vi "TagWrite.vi"(7 "LabVIEW Web Service Request":refnum<class "Web Request.lvclass">, 10 "tagName":string, 11 "type":string) -> ()   [LabVIEW 2013]
doc: "TagWrite assigns the given value to the tag specified. Specifying the type isn't required, but results in slightly faster performance."
uses:
  <vilib>/wsapi/Web Request.lvclass
  <vilib>/NI/Tag Bus/tag/Data Type.ctl
  <vilib>/NI/Tag Bus/table/data polymorphs/write one/write Double.vi
  <vilib>/NI/Tag Bus/table/data polymorphs/write one/write Single.vi
  <vilib>/NI/Tag Bus/table/data polymorphs/write one/write I64.vi
  <vilib>/NI/Tag Bus/table/data polymorphs/write one/write I32.vi
  <vilib>/NI/Tag Bus/table/data polymorphs/write one/write I16.vi
  <vilib>/NI/Tag Bus/table/data polymorphs/write one/write I8.vi
  <vilib>/NI/Tag Bus/table/data polymorphs/write one/write U64.vi
  <vilib>/NI/Tag Bus/table/data polymorphs/write one/write U32.vi
  <vilib>/NI/Tag Bus/table/data polymorphs/write one/write U16.vi
  <vilib>/NI/Tag Bus/table/data polymorphs/write one/write U8.vi
  <vilib>/NI/Tag Bus/table/data polymorphs/write one/write String.vi
  <vilib>/NI/Tag Bus/table/data polymorphs/write one/write Boolean.vi
  <vilib>/NI/TagWebClient/API/tagweb client API.lvlib
  <vilib>/NI/Tag Bus/tag/tag descriptor.lvclass
  <vilib>/NI/Tag Bus/table/data table.lvlib
  <vilib>/NI/Tag Bus/dictionary/data dictionary.lvclass
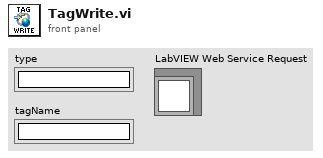
[diagram p1: front panel]
types:
  T1 = typedef "tag bus.lvlib/tag descriptor.lvclass/Data Type.ctl" = enum16{"Double", "Single", "I64", "I32", "I16", "I8", "U64", "U32", "U16", "U8", "Boolean", "String", "Array of Double", "Array of Single", "Array of I64", "Array of I32", "Array of I16", "Array of I8", "Array of U64", "Array of U32", "Array of U16", "Array of U8", "Array of Boolean", "Array of String"}
  T2 = typedef "tag bus.lvlib/data table.lvlib/data table.ctl" = cluster{"Double":dbl[], "Single":sgl[], "I64":i64[], "I32":i32[], "I16":i16[], "I8":i8[], "U64":u64[], "U32":u32[], "U16":u16[], "U8":u8[], "Boolean":bool[], "String":string[], "Array of Double":cluster{"DBL Array":dbl[]}[], "Array of Single":cluster{"SGL Array":sgl[]}[], "Array of I64":cluster{"I64 Array":i64[]}[], "Array of I32":cluster{"I32 Array":i32[]}[], "Array of I16":cluster{"I16 Array":i16[]}[], "Array of I8":cluster{"I8 Array":i8[]}[], "Array of U64":cluster{"U64 Array":u64[]}[], "Array of U32":cluster{"U32 Array":u32[]}[], "Array of U16":cluster{"U16 Array":u16[]}[], "Array of U8":cluster{"U8 Array":u8[]}[], "Array of Boolean":cluster{"Boolean Array":bool[]}[], "Array of String":cluster{"String Array":string[]}[]}
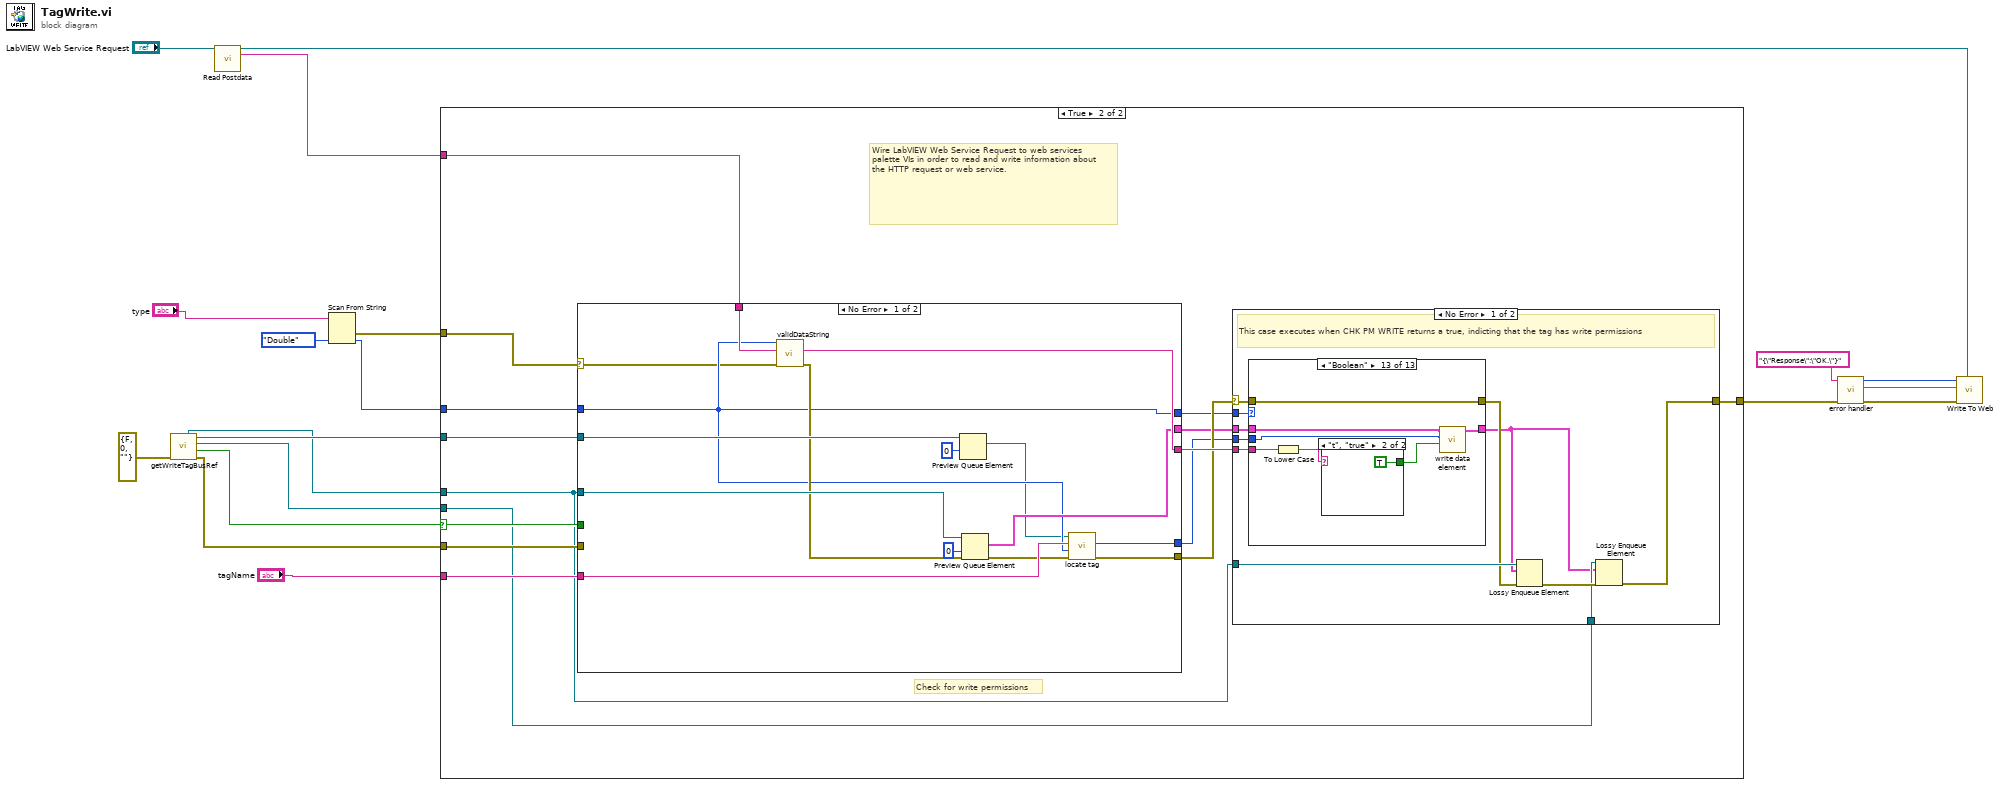
[diagram p0: block diagram]
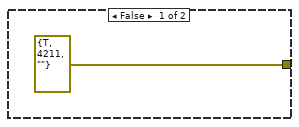
[diagram p2: hidden frame]
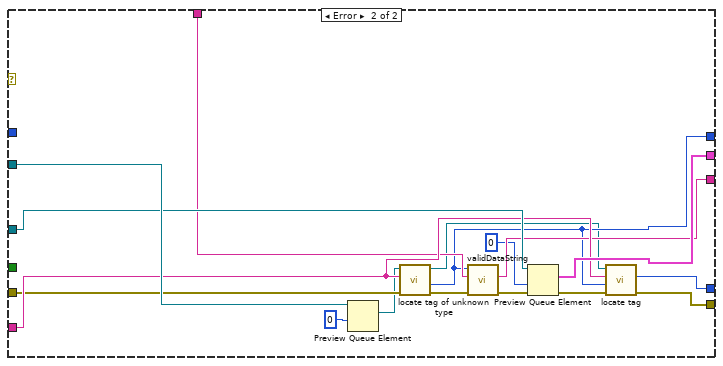
[diagram p3: hidden frame]
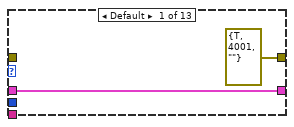
[diagram p4: hidden frame]
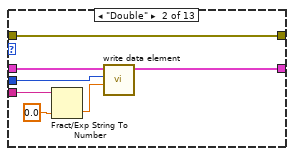
[diagram p5: hidden frame]
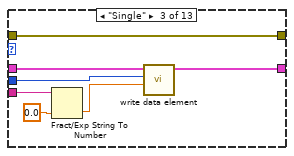
[diagram p6: hidden frame]
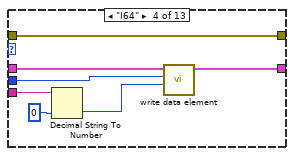
[diagram p7: hidden frame]
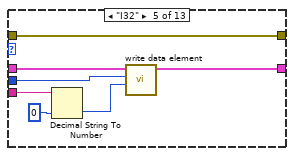
[diagram p8: hidden frame]
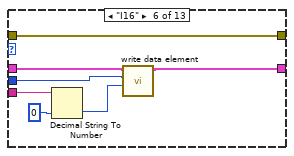
[diagram p9: hidden frame]
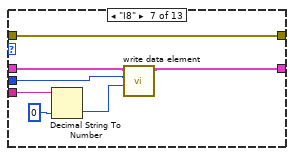
[diagram p10: hidden frame]
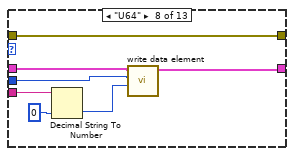
[diagram p11: hidden frame]
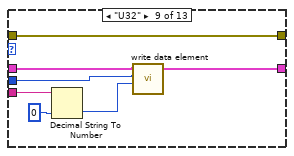
[diagram p12: hidden frame]
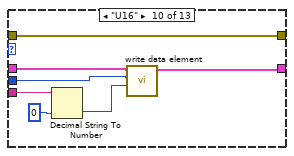
[diagram p13: hidden frame]
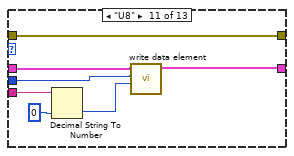
[diagram p14: hidden frame]
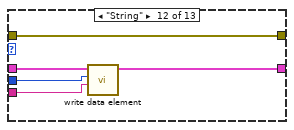
[diagram p15: hidden frame]
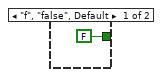
[diagram p16: hidden frame]
diagram:
  n1 = call "getWriteTagBusRef.vi"("error in"=errorcluster {"status"=FALSE, "code"=0, "source"=""} ("error in (no error)")) -> ("error out"=w14:errorcluster, "valid references"=w5:bool, "write tx data table"=w9:refnum<queue>, "write data dictionary"=w15:refnum<queue>, "actual write data table"=w10:refnum<queue>)  [unwired: 6 in]
  n2 = call <vilib>:"Read Postdata.vi"("LabVIEW Web Service Request"="LabVIEW Web Service Request") -> ("LabVIEW Web Service Request out"=w1:refnum<class "Web Request.lvclass">, "postdata"=w4:string)  [unwired: 12 in, 1 out]
  n3 = Scan From String(input string="type", default 1=Data_Type."Double" ("data type")) -> (error out=w12:errorcluster, output 1=w11:T1)  [unwired: 3 in, 2 out]
  n4 = case shown="True" w5 {
    selector: w5 -> [_ w23]
    tunnel: [errorcluster {"status"=TRUE, "code"=4211, "source"=""} ("error IO") w35] -> w18
    tunnel: w15 -> [_ w34]
    tunnel: w14 -> [_ w28]
    tunnel: w4 -> [_ w27]
    tunnel: "tagName" -> [_ w26]
    tunnel: w12 -> [_ w25]
    tunnel: w11 -> [_ w24]
    tunnel: w10 -> [_ w21]
    tunnel: w9 -> [_ w22]
    frame False {
    }
    frame True {
      # "Check for write permissions"
      # "Wire LabVIEW Web Service Request to web services palette VIs in order to read and write information about the HTTP request or web service."
      n5 = case shown="No Error" w25 {
        selector: w25 -> [w36 _]
        tunnel: w27 -> [w50 w61]
        tunnel: w34 -> [w49 w67]
        tunnel: w21 -> [w48 w66]
        tunnel: [w47 w60] -> w33
        tunnel: w23 -> [_ _]
        tunnel: w26 -> [w45 w62]
        tunnel: [w44 w65] -> w32
        tunnel: [w41 w59] -> w31
        tunnel: [w43 w64] -> w30
        tunnel: [w42 w63] -> w29
        tunnel: w28 -> [_ w58]
        tunnel: w24 -> [w41 _]
        frame No Error {
          n6 = call "validDataString.vi"("error in (no error)"=w36, "value in"=w50, "data type"=w41) -> ("error out"=w46:errorcluster, "value out"=w47:string)  [unwired: 6 in, 1 out]
          n7 = Preview Queue Element(queue=w49, timeout in ms (-1)=0) -> (element=w37:refnum<class "data dictionary.lvclass">)  [unwired: 1 in, 3 out]
          n8 = Preview Queue Element(queue=w48, timeout in ms (-1)=0, error in (no error)=w46) -> (element=w42:T2, error out=w39:errorcluster)  [unwired: 2 out]
          n9 = call <vilib>:"locate tag.vi"("error in"=w39, "data type"=w41, "name"=w45, "data dictionary in"=w37) -> ("error out"=w44:errorcluster, "index"=w43:i32)  [unwired: 5 in, 1 out]
        }
        frame Error {
          n10 = Preview Queue Element(queue=w67, timeout in ms (-1)=0) -> (element=w51:refnum<class "data dictionary.lvclass">)  [unwired: 1 in, 3 out]
          n11 = call <vilib>:"locate tag of unknown type.vi"("error in"=w58, "name"=w62, "data dictionary in"=w51) -> ("error out"=w53:errorcluster, "data type"=w59:T1, "data dictionary out"=w52:refnum<class "data dictionary.lvclass">)  [unwired: 5 in, 1 out]
          n12 = call "validDataString.vi"("error in (no error)"=w53, "value in"=w61, "data type"=w59) -> ("error out"=w54:errorcluster, "value out"=w60:string)  [unwired: 6 in, 1 out]
          n13 = Preview Queue Element(queue=w66, timeout in ms (-1)=0, error in (no error)=w54) -> (element=w63:T2, error out=w56:errorcluster)  [unwired: 2 out]
          n14 = call <vilib>:"locate tag.vi"("error in"=w56, "data type"=w59, "name"=w62, "data dictionary in"=w52) -> ("error out"=w65:errorcluster, "index"=w64:i32)  [unwired: 5 in, 1 out]
        }
      }
      n15 = case shown="No Error" w32 {
        selector: w32 -> [w74 w165]
        tunnel: w33 -> [w78 _]
        tunnel: w30 -> [w77 _]
        tunnel: [w70 w165] -> w35
        tunnel: w31 -> [w76 _]
        tunnel: w29 -> [w75 _]
        tunnel: w21 -> [w73 _]
        tunnel: w22 -> [w69 _]
        frame No Error {
          # "This case executes when CHK PM WRITE returns a true, indicting that the tag has write permissions"
          n16 = case shown="\"Boolean\"" w76 {
            tunnel: w77 -> [_ w84 w89 w96 w103 w110 w117 w125 w132 w138 w145 w153 w157]
            tunnel: [errorcluster {"status"=TRUE, "code"=4001, "source"=""} ("error out") w82 w92 w99 w106 w113 w120 w127 w134 w141 w148 w155 w160] -> w72
            tunnel: w78 -> [_ w87 w94 w101 w108 w115 w122 w129 w136 w143 w150 w152 w162]
            tunnel: w75 -> [w79 w85 w91 w98 w104 w111 w118 w126 w133 w140 w146 w154 w159]
            tunnel: w74 -> [_ w82 w92 w99 w106 w113 w120 w127 w134 w141 w148 w155 w160]
            tunnel: [w79 w81 w90 w97 w105 w112 w119 w123 w130 w139 w147 w151 w158] -> w68
            frame Default {
            }
            frame "Double" {
              n17 = Fract/Exp String To Number(string=w87, default (0 dbl)=0.0 ("Value")) -> (number=w83:dbl)  [unwired: 2 in, 1 out]
              n18 = call-poly <vilib>:"write data element.vi"("value"=w83, "index"=w84, "data table in"=w85) -> ("data table out"=w81:T2)  [unwired: 8 in]
            }
            frame "Single" {
              n19 = Fract/Exp String To Number(string=w94, default (0 dbl)=sgl 0.0 ("Value")) -> (number=w88:sgl)  [unwired: 2 in, 1 out]
              n20 = call-poly <vilib>:"write data element.vi"("value"=w88, "index"=w89, "data table in"=w91) -> ("data table out"=w90:T2)  [unwired: 8 in]
            }
            frame "I64" {
              n21 = Decimal String To Number(string=w101, default (0L)=i64 0 ("Value")) -> (number=w95:i64)  [unwired: 1 in, 1 out]
              n22 = call-poly <vilib>:"write data element.vi"("value"=w95, "index"=w96, "data table in"=w98) -> ("data table out"=w97:T2)  [unwired: 8 in]
            }
            frame "I32" {
              n23 = Decimal String To Number(string=w108, default (0L)=0 ("Value")) -> (number=w102:i32)  [unwired: 1 in, 1 out]
              n24 = call-poly <vilib>:"write data element.vi"("value"=w102, "index"=w103, "data table in"=w104) -> ("data table out"=w105:T2)  [unwired: 8 in]
            }
            frame "I16" {
              n25 = Decimal String To Number(string=w115, default (0L)=i16 0 ("Value")) -> (number=w109:i16)  [unwired: 1 in, 1 out]
              n26 = call-poly <vilib>:"write data element.vi"("value"=w109, "index"=w110, "data table in"=w111) -> ("data table out"=w112:T2)  [unwired: 8 in]
            }
            frame "I8" {
              n27 = Decimal String To Number(string=w122, default (0L)=i8 0 ("Value")) -> (number=w116:i8)  [unwired: 1 in, 1 out]
              n28 = call-poly <vilib>:"write data element.vi"("value"=w116, "index"=w117, "data table in"=w118) -> ("data table out"=w119:T2)  [unwired: 8 in]
            }
            frame "U64" {
              n29 = Decimal String To Number(string=w129, default (0L)=u64 0 ("Value")) -> (number=w124:u64)  [unwired: 1 in, 1 out]
              n30 = call-poly <vilib>:"write data element.vi"("value"=w124, "index"=w125, "data table in"=w126) -> ("data table out"=w123:T2)  [unwired: 8 in]
            }
            frame "U32" {
              n31 = Decimal String To Number(string=w136, default (0L)=u32 0 ("Value")) -> (number=w131:u32)  [unwired: 1 in, 1 out]
              n32 = call-poly <vilib>:"write data element.vi"("value"=w131, "index"=w132, "data table in"=w133) -> ("data table out"=w130:T2)  [unwired: 8 in]
            }
            frame "U16" {
              n33 = Decimal String To Number(string=w143, default (0L)=u16 0 ("Value")) -> (number=w137:u16)  [unwired: 1 in, 1 out]
              n34 = call-poly <vilib>:"write data element.vi"("value"=w137, "index"=w138, "data table in"=w140) -> ("data table out"=w139:T2)  [unwired: 8 in]
            }
            frame "U8" {
              n35 = Decimal String To Number(string=w150, default (0L)=u8 0 ("Value")) -> (number=w144:u8)  [unwired: 1 in, 1 out]
              n36 = call-poly <vilib>:"write data element.vi"("value"=w144, "index"=w145, "data table in"=w146) -> ("data table out"=w147:T2)  [unwired: 8 in]
            }
            frame "String" {
              n37 = call-poly <vilib>:"write data element.vi"("value"=w152, "index"=w153, "data table in"=w154) -> ("data table out"=w151:T2)  [unwired: 8 in]
            }
            frame "Boolean" {
              n38 = To Lower Case(string=w162) -> (all lower case string=w161:string)
              n39 = case shown="\"t\", \"true\"" w161 {
                tunnel: [FALSE ("Value") TRUE ("Value")] -> w156
                frame "f", "false", Default {
                }
                frame "t", "true" {
                }
              }
              n40 = call-poly <vilib>:"write data element.vi"("value"=w156, "index"=w157, "data table in"=w159) -> ("data table out"=w158:T2)  [unwired: 8 in]
            }
          }
          n41 = Lossy Enqueue Element(queue=w73, element=w68, error in (no error)=w72) -> (error out=w71:errorcluster)  [unwired: 3 out]
          n42 = Lossy Enqueue Element(queue=w69, element=w68, error in (no error)=w71) -> (error out=w70:errorcluster)  [unwired: 3 out]
        }
        frame Error {
          # "This case executes when CHK PM WRITE returns a false, indicating that the tag does not have write permissions"
        }
      }
    }
  }
  n43 = call "error handler.vi"("error in (no error)"=w18, "Success Message"="{\"Response\":\"OK.\"}" ("response string")) -> ("error out"=w8:errorcluster, "Response String"=w6:string, "Response Code"=w7:i32)  [unwired: 7 in]
  n44 = call <vilib>:"Write To Web.vi"("Web Request in"=w1, "error in"=w8, "Response String"=w6, "Response Code"=w7) -> ()  [unwired: 8 in]
